vi "AnalysisDisplay_171213.vi"(0 "TraceLength":dbl, 1 "Segments":bool, 2 "FullTrack":bool, 3 "FulltrackonBackgroundSegments":picture, 4 "BackgroundSegments":picture, 5 "NormalMouseBackground":picture, 6 "X":i32, 7 "Y":i32, 8 "i":i32, 9 "X in":i32[](array[numeric]), 10 "Angle":dbl, 11 "Y in":i32[](array[numeric]), 14 "FulltrackonNormalMouseBackground":picture) -> (12 "X out":i32[](array[numeric]), 13 "Y out":i32[](array[numeric]), 19 "AnalysisDisplayOutput":picture)   [LabVIEW 2016]
uses:
  Globaltracker.vi
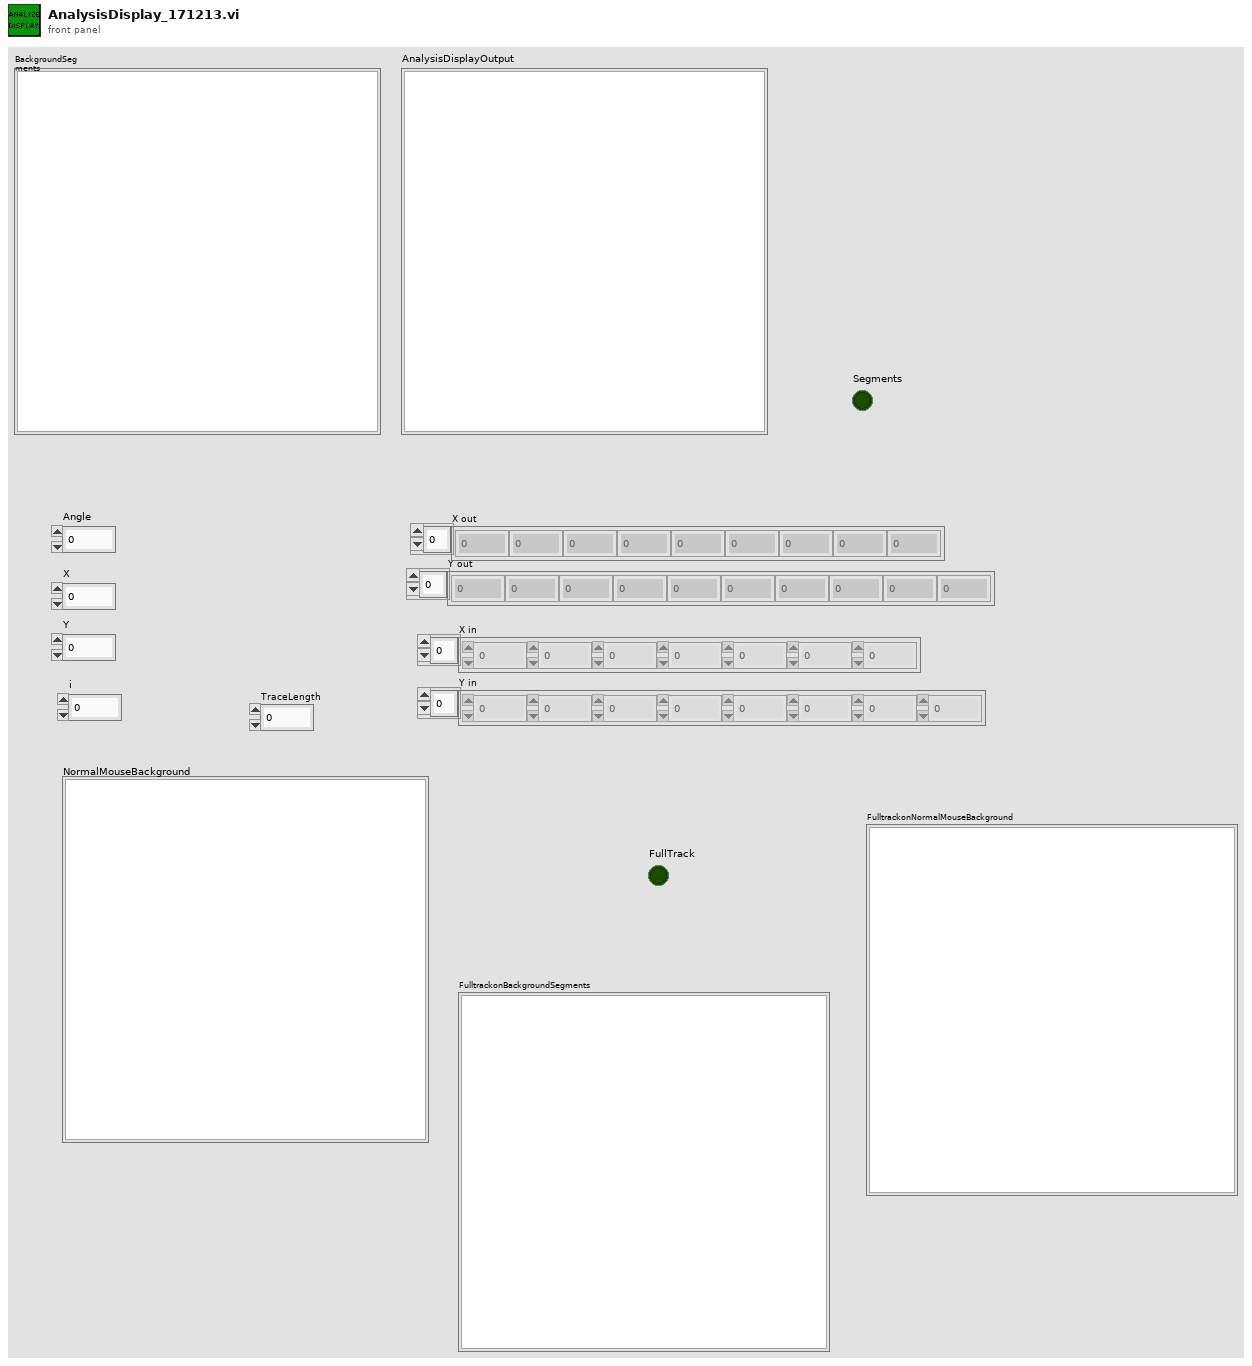
[diagram p1: front panel]
types:
  T1 = typedef "imagedata.ctl" = cluster{"image type":i32, "image depth":i32, "image":u8[], "mask":u8[], "colors":u32[], "Rectangle":cluster{"left":i16, "top":i16, "right":i16, "bottom":i16}}
  T2 = cluster{"left":i16, "top":i16, "right":i16, "bottom":i16}
  T3 = cluster{"image type":i32, "image depth":i32, "image":u8[], "mask":u8[], "colors":u32[], cluster{i32, i32, i32, i32}}
  T4 = cluster{"Width":u16, "Style":enum32{"Solid", "Dash", "Dot", "DashDot", "DashDotDot"}}
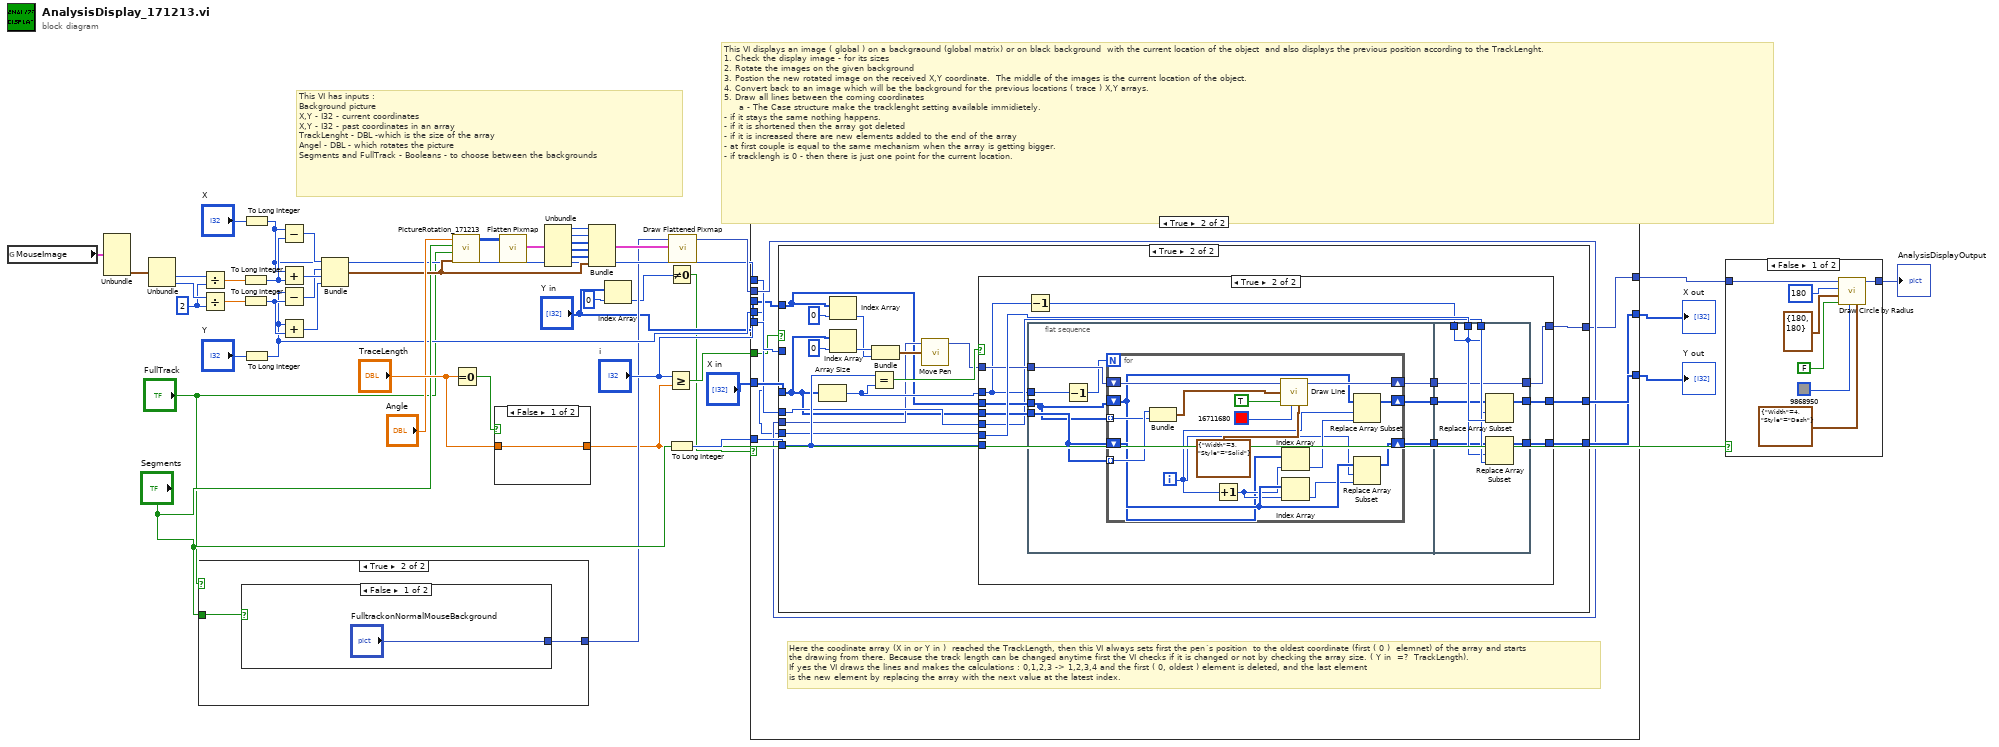
[diagram p0: block diagram]
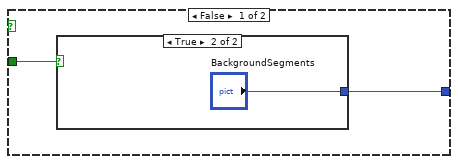
[diagram p2: hidden frame]
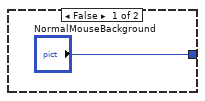
[diagram p3: hidden frame]
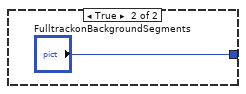
[diagram p4: hidden frame]
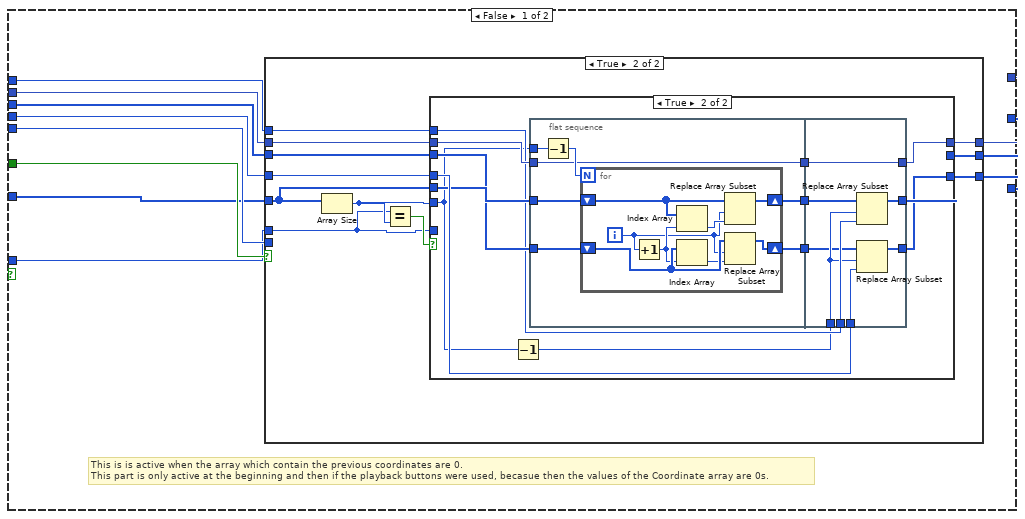
[diagram p5: hidden frame]
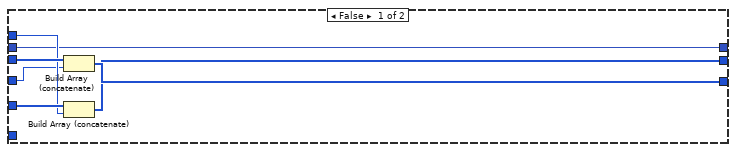
[diagram p6: hidden frame]
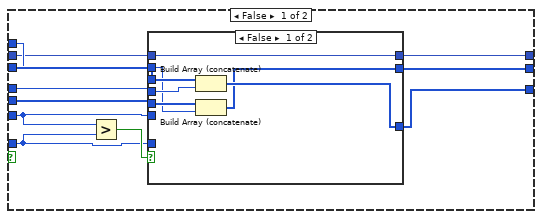
[diagram p7: hidden frame]
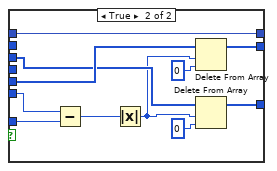
[diagram p8: hidden frame]
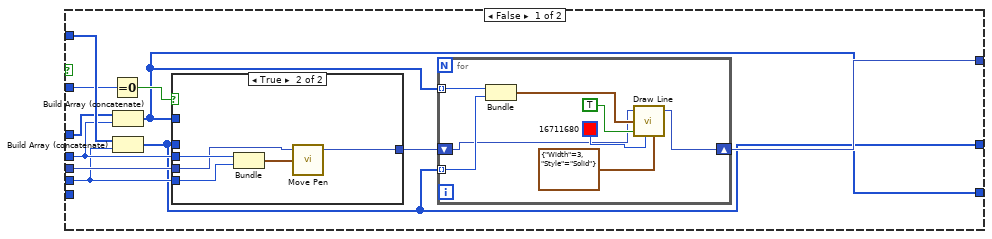
[diagram p9: hidden frame]
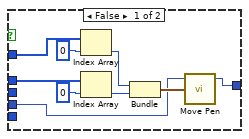
[diagram p10: hidden frame]
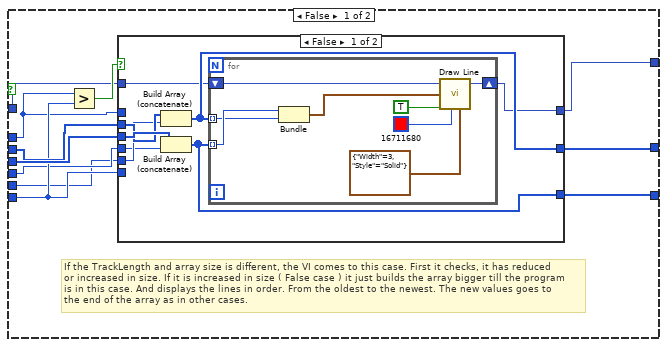
[diagram p11: hidden frame]
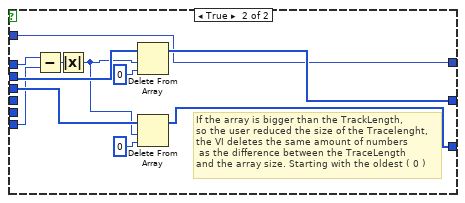
[diagram p12: hidden frame]
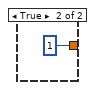
[diagram p13: hidden frame]
diagram:
  w19 = i16 2 ("y")
  # "This VI displays an image ( global ) on a backgraound (global matrix) or on black background  with the current location of the object  and also displays the previous position according to the TrackLenght.\n1. Check the display image - for its sizes\n2. Rotate the images on the given background\n3. Postion the new rotated image on the received X,Y coordinate.  The middle of the images is the current location of the object.\n4. Convert back to an image which will be the background for the previous locations ( trace ) X,Y arrays. \n5. Draw all lines between the coming coordinates \n     a - The Case structure make the tracklenght setting available immidietely. \n- if it stays the same nothing happens.\n- if it is shortened then the array got deleted\n- if it is increased there are new elements added to the end of the array\n- at first couple is equal to the same mechanism when the array is getting bigger.\n- if tracklengh is 0 - then there is just one point for the current location."
  # "This VI has inputs : \nBackground picture\nX,Y - I32 - current coordinates \nX,Y - I32 - past coordinates in an array \nTrackLenght - DBL -which is the size of the array\nAngel - DBL - which rotates the picture\nSegments and FullTrack - Booleans - to choose between the backgrounds"
  n1 = global read "Globaltracker.vi" "MouseImage"() -> (w23:T1)
  n2 = Unbundle(w23) -> ("Rectangle"=w22:T2)  [unwired: 5 out]
  n3 = Unbundle(w22) -> ("right"=w21:i16, "bottom"=w20:i16)  [unwired: 2 out]
  n4 = case shown="True" "FullTrack" {
    tunnel: "Segments" -> [w48 w52]
    tunnel: [w47 w51] -> w8
    frame False {
      n5 = case shown="True" w48 {
        tunnel: ["NormalMouseBackground" "BackgroundSegments"] -> w47
        frame False {
        }
        frame True {
        }
      }
    }
    frame True {
      n6 = case shown="False" w52 {
        tunnel: ["FulltrackonNormalMouseBackground" "FulltrackonBackgroundSegments"] -> w51
        frame False {
        }
        frame True {
        }
      }
    }
  }
  n7 = Divide(x=w21, y=w19) -> (x/y=w18:dbl)
  n8 = Divide(x=w20, y=w19) -> (x/y=w17:dbl)
  n9 = To Long Integer(number=w18) -> (32bit integer=w16:i32)
  n10 = To Long Integer(number=w17) -> (32bit integer=w15:i32)
  n11 = To Long Integer(number="X") -> (32bit integer=w10:i32)
  n12 = To Long Integer(number="Y") -> (32bit integer=w9:i32)
  n13 = Subtract(x=w10, y=w16) -> (x-y=w39:i32)
  n14 = Add(x=w10, y=w16) -> (x+y=w38:i32)
  n15 = Subtract(x=w9, y=w15) -> (x-y=w36:i32)
  n16 = Add(x=w9, y=w15) -> (x+y=w37:i32)
  n17 = Bundle(w39, w36, w38, w37) -> (w28:cluster{i32, i32, i32, i32})  [unwired: 1 in]
  n18 = call "PictureRotation_171213.vi"("Cluster"=w28, "FullTrack"="FullTrack", "Segments"="Segments", "Angle"="Angle") -> ("Array"=w14:u32[][])  [unwired: 7 in]
  n19 = Equal To 0?(x="TraceLength") -> (x = 0?=w45:bool)
  n20 = case shown="False" w45 {
    tunnel: "TraceLength" -> [w55 _]
    tunnel: [w55 1] -> w7
    frame False {
    }
    frame True {
    }
  }
  n21 = call <vilib>:"Flatten Pixmap.vi"("24-bit pixmap"=w14) -> ("image data"=w34:T1)  [unwired: 10 in]
  n22 = Unbundle(w34) -> ("image type"=w33:i32, "image depth"=w32:i32, "image"=w31:u8[], "mask"=w30:u8[], "colors"=w29:u32[])  [unwired: 1 out]
  n23 = Bundle("image type"=w33, "image depth"=w32, "image"=w31, "mask"=w30, "colors"=w29, w28) -> (w25:T3)  [unwired: 1 in]
  n24 = Index Array(array="Y in", index=0) -> (element=w4:i32)
  n25 = Greater Or Equal?(x="i", y=w7) -> (x >= y?=w6:bool)
  n26 = Not Equal To 0?(x=w4) -> (x != 0?=w3:bool)
  n27 = To Long Integer(number=w7) -> (32bit integer=w43:i32)
  n28 = call <vilib>:"Draw Flattened Pixmap.vi"("image data"=w25, "picture"=w8) -> ("new picture"=w24:picture)  [unwired: 7 in]
  n29 = case shown="True" w3 {
    tunnel: "i" -> [w66 w161]
    tunnel: w43 -> [w65 w160]
    tunnel: "X in" -> [w61 w159]
    tunnel: [w57 w158] -> w41
    tunnel: [w58 w157] -> w40
    tunnel: w24 -> [w60 w156]
    tunnel: [w59 w155] -> w13
    tunnel: w10 -> [w63 w154]
    tunnel: w9 -> [w64 w153]
    tunnel: "Y in" -> [w62 w152]
    tunnel: w6 -> [w67 w151]
    frame False {
      # "This is is active when the array which contain the previous coordinates are 0. \nThis part is only active at the beginning and then if the playback buttons were used, becasue then the values of the Coordinate array are 0s."
      n30 = case shown="True" w67 {
        tunnel: [w68 w84] -> w59
        tunnel: w66 -> [_ _]
        tunnel: w65 -> [_ w81]
        tunnel: w64 -> [w71 w80]
        tunnel: [w69 w78] -> w58
        tunnel: [w70 w85] -> w57
        tunnel: w62 -> [w74 w77]
        tunnel: w61 -> [w73 w76]
        tunnel: w63 -> [w72 w79]
        tunnel: w60 -> [w68 w75]
        frame False {
          n31 = Build Array (concatenate)(w74, w71) -> (w70:i32[])
          n32 = Build Array (concatenate)(w73, w72) -> (w69:i32[])
        }
        frame True {
          n33 = Array Size(array=w76) -> (size(s)=w82:i32)
          n34 = Equal?(x=w81, y=w82) -> (x = y?=w83:bool)
          n35 = case shown="True" w83 {
            tunnel: [w95 w127] -> w78
            tunnel: [w94 w126] -> w85
            tunnel: w80 -> [w86 w125]
            tunnel: w76 -> [w93 w124]
            tunnel: w77 -> [w92 w123]
            tunnel: w75 -> [w88 w122]
            tunnel: [w87 w118] -> w84
            tunnel: w82 -> [w90 w117]
            tunnel: w81 -> [w91 _]
            tunnel: w79 -> [w89 w121]
            frame False {
              n36 = Greater?(x=w90, y=w91) -> (0:w96:bool)
              n37 = case shown="False" w96 {
                tunnel: [w98 w114] -> w95
                tunnel: [w99 w113] -> w94
                tunnel: w93 -> [w103 w112]
                tunnel: w92 -> [w102 w111]
                tunnel: w90 -> [_ w110]
                tunnel: w91 -> [_ w106]
                tunnel: w86 -> [w101 _]
                tunnel: w89 -> [w100 _]
                tunnel: w88 -> [w97 w107]
                tunnel: [w97 w107] -> w87
                frame False {
                  n38 = Build Array (concatenate)(w102, w101) -> (w99:i32[])
                  n39 = Build Array (concatenate)(w103, w100) -> (w98:i32[])
                }
                frame True {
                  n40 = Subtract(x=w110, y=w106) -> (x-y=w109:i32)
                  n41 = Absolute Value(x=w109) -> (abs(x)=w108:i32)
                  n42 = Delete From Array(array=w112, length=w108, index=0) -> (array with subset deleted=w114:i32[])  [unwired: 1 out]
                  n43 = Delete From Array(array=w111, length=w108, index=0) -> (array with subset deleted=w113:i32[])  [unwired: 1 out]
                }
              }
            }
            frame True {
              n44 = Decrement(x=w117) -> (x-1=w120:i32)
              n45 = flat-sequence {
                tunnel: w124 -> [w134]
                tunnel: w123 -> [w133]
                tunnel: w122 -> [w128]
                tunnel: [w128] -> w119
                tunnel: w117 -> [w132]
                tunnel: [w130] -> w116
                tunnel: [w129] -> w115
                tunnel: [w150] -> w127
                tunnel: [w149] -> w126
                tunnel: w125 -> [w148]
                tunnel: w121 -> [w147]
                tunnel: w120 -> [w146]
                tunnel: w119 -> [w145]
                tunnel: [w145] -> w118
                tunnel: w116 -> [w144]
                tunnel: w115 -> [w143]
                frame #0 {
                  n46 = Decrement(x=w132) -> (x-1=w131:i32)
                  n47 = for {
                    N: w131 -> [_]
                    shift-right: [w136] -> w130
                    shift-left: w134 -> [w142]
                    shift-right: [w135] -> w129
                    shift-left: w133 -> [w141]
                    i -> [w137]
                    n48 = Increment(x=w137) -> (x+1=w140:i32)
                    n49 = Index Array(array=w142, index=w140) -> (element=w139:i32)
                    n50 = Index Array(array=w141, index=w140) -> (element=w138:i32)
                    n51 = Replace Array Subset(array=w142, new element=w139, index=w137) -> (w136:i32[])
                    n52 = Replace Array Subset(array=w141, new element=w138, index=w137) -> (w135:i32[])
                  }
                }
                frame #1 {
                  n53 = Replace Array Subset(array=w144, new element=w147, index=w146) -> (w150:i32[])
                  n54 = Replace Array Subset(array=w143, new element=w148, index=w146) -> (w149:i32[])
                }
              }
            }
          }
        }
      }
    }
    frame True {
      # "Here the coodinate array (X in or Y in )  reached the TrackLength, then this VI always sets first the pen´s position  to the oldest coordinate (first ( 0 )  elemnet) of the array and starts \nthe drawing from there. Because the track length can be changed anytime first the VI checks if it is changed or not by checking the array size. ( Y in  =?  TrackLength).\nIf yes the VI draws the lines and makes the calculations : 0,1,2,3 -> 1,2,3,4 and the first ( 0, oldest ) element is deleted, and the last element\nis the new element by replacing the array with the next value at the latest index."
      n55 = case shown="True" w151 {
        tunnel: [w170 w210] -> w155
        tunnel: w161 -> [w165 _]
        tunnel: w160 -> [_ w207]
        tunnel: w153 -> [w167 w206]
        tunnel: [w162 w204] -> w157
        tunnel: [w163 w211] -> w158
        tunnel: w152 -> [w172 w196]
        tunnel: w159 -> [w171 w195]
        tunnel: w154 -> [w169 w205]
        tunnel: w156 -> [w168 w198]
        frame False {
          n56 = Equal To 0?(x=w165) -> (x = 0?=w166:bool)
          n57 = Build Array (concatenate)(w171, w169) -> (w162:i32[])
          n58 = Build Array (concatenate)(w172, w167) -> (w163:i32[])
          n59 = case shown="True" w166 {
            tunnel: w169 -> [_ w186]
            tunnel: w168 -> [w179 w185]
            tunnel: w167 -> [_ w184]
            tunnel: [w180 w182] -> w164
            tunnel: w163 -> [w178 _]
            tunnel: w162 -> [w177 _]
            frame False {
              n60 = Index Array(array=w177, index=0) -> (element=w174:i32)
              n61 = Index Array(array=w178, index=0) -> (element=w173:i32)
              n62 = Bundle(w174, w173) -> (w181:cluster{i32, i32})  [unwired: 1 in]
              n63 = call <vilib>:"Move Pen.vi"("new position"=w181, "picture"=w179) -> ("new picture"=w180:picture)  [unwired: 3 in]
            }
            frame True {
              n64 = Bundle(w186, w184) -> (w183:cluster{i32, i32})  [unwired: 1 in]
              n65 = call <vilib>:"Move Pen.vi"("new position"=w183, "picture"=w185) -> ("new picture"=w182:picture)  [unwired: 3 in]
            }
          }
          n66 = for {
            tunnel: w162 -> [w194] mode=indexing
            tunnel: w163 -> [w193] mode=indexing
            shift-right: [w188] -> w170
            shift-left: w164 -> [w187]
            n67 = Bundle(w194, w193) -> (w189:cluster{i32, i32})  [unwired: 1 in]
            n68 = call <vilib>:"Draw Line.vi"("picture"=w187, "end point"=w189, "absolute coordinates?(T)"=TRUE, "color(black)"=u32 16711680, "pen"=T4 {"Width"=3, "Style"=enum."Solid"}) -> ("new picture"=w188:picture)  [unwired: 4 in]
          }
        }
        frame True {
          n69 = Array Size(array=w195) -> (size(s)=w208:i32)
          n70 = Index Array(array=w196, index=0) -> (element=w201:i32)
          n71 = Index Array(array=w195, index=0) -> (element=w202:i32)
          n72 = Equal?(x=w207, y=w208) -> (x = y?=w209:bool)
          n73 = Bundle(w202, w201) -> (w203:cluster{i32, i32})  [unwired: 1 in]
          n74 = call <vilib>:"Move Pen.vi"("new position"=w203, "picture"=w198) -> ("new picture"=w197:picture)  [unwired: 3 in]
          n75 = case shown="True" w209 {
            tunnel: [w221 w262] -> w204
            tunnel: [w220 w261] -> w211
            tunnel: w206 -> [w212 w260]
            tunnel: w195 -> [w219 w259]
            tunnel: w196 -> [w218 w258]
            tunnel: w197 -> [w214 w257]
            tunnel: [w213 w253] -> w210
            tunnel: w208 -> [w216 w252]
            tunnel: w207 -> [w217 _]
            tunnel: w205 -> [w215 w256]
            frame False {
              # "If the TrackLength and array size is different, the VI comes to this case. First it checks, it has reduced\nor increased in size. If it is increased in size ( False case ) it just builds the array bigger till the program\nis in this case. And displays the lines in order. From the oldest to the newest. The new values goes to\nthe end of the array as in other cases."
              n76 = Greater?(x=w216, y=w217) -> (0:w222:bool)
              n77 = case shown="False" w222 {
                tunnel: [w225 w249] -> w221
                tunnel: [w226 w248] -> w220
                tunnel: w219 -> [w230 w247]
                tunnel: w218 -> [w229 w246]
                tunnel: w216 -> [_ w245]
                tunnel: w217 -> [_ w241]
                tunnel: w212 -> [w228 _]
                tunnel: w215 -> [w227 _]
                tunnel: w214 -> [w224 w242]
                tunnel: [w223 w242] -> w213
                frame False {
                  n78 = Build Array (concatenate)(w229, w228) -> (w226:i32[])
                  n79 = Build Array (concatenate)(w230, w227) -> (w225:i32[])
                  n80 = for {
                    tunnel: w225 -> [w238] mode=indexing
                    tunnel: w226 -> [w237] mode=indexing
                    shift-right: [w231] -> w223
                    shift-left: w224 -> [w233]
                    n81 = Bundle(w238, w237) -> (w232:cluster{i32, i32})  [unwired: 1 in]
                    n82 = call <vilib>:"Draw Line.vi"("picture"=w233, "end point"=w232, "absolute coordinates?(T)"=TRUE, "color(black)"=u32 16711680, "pen"=T4 {"Width"=3, "Style"=enum."Solid"}) -> ("new picture"=w231:picture)  [unwired: 4 in]
                  }
                }
                frame True {
                  # "If the array is bigger than the TrackLength,\nso the user reduced the size of the Tracelenght,\nthe VI deletes the same amount of numbers\n as the difference between the TraceLength \nand the array size. Starting with the oldest ( 0 )"
                  n83 = Subtract(x=w245, y=w241) -> (x-y=w244:i32)
                  n84 = Absolute Value(x=w244) -> (abs(x)=w243:i32)
                  n85 = Delete From Array(array=w246, length=w243, index=0) -> (array with subset deleted=w248:i32[])  [unwired: 1 out]
                  n86 = Delete From Array(array=w247, length=w243, index=0) -> (array with subset deleted=w249:i32[])  [unwired: 1 out]
                }
              }
            }
            frame True {
              n87 = Decrement(x=w252) -> (x-1=w255:i32)
              n88 = flat-sequence {
                tunnel: w259 -> [w268]
                tunnel: w258 -> [w267]
                tunnel: w257 -> [w270]
                tunnel: [w269] -> w254
                tunnel: w252 -> [w266]
                tunnel: [w264] -> w251
                tunnel: [w263] -> w250
                tunnel: [w294] -> w262
                tunnel: [w293] -> w261
                tunnel: w260 -> [w292]
                tunnel: w256 -> [w291]
                tunnel: w255 -> [w290]
                tunnel: w254 -> [w289]
                tunnel: [w289] -> w253
                tunnel: w251 -> [w288]
                tunnel: w250 -> [w287]
                frame #0 {
                  n89 = Decrement(x=w266) -> (x-1=w265:i32)
                  n90 = for {
                    N: w265 -> [_]
                    tunnel: w268 -> [w286] mode=indexing
                    tunnel: w267 -> [w285] mode=indexing
                    shift-right: [w280] -> w269
                    shift-left: w270 -> [w282]
                    shift-right: [w275] -> w264
                    shift-left: w268 -> [w279]
                    shift-right: [w274] -> w263
                    shift-left: w267 -> [w273]
                    i -> [w272]
                    n91 = Bundle(w286, w285) -> (w281:cluster{i32, i32})  [unwired: 1 in]
                    n92 = Increment(x=w272) -> (x+1=w278:i32)
                    n93 = call <vilib>:"Draw Line.vi"("picture"=w282, "end point"=w281, "absolute coordinates?(T)"=TRUE, "color(black)"=u32 16711680, "pen"=T4 {"Width"=3, "Style"=enum."Solid"}) -> ("new picture"=w280:picture)  [unwired: 4 in]
                    n94 = Index Array(array=w273, index=w278) -> (element=w276:i32)
                    n95 = Index Array(array=w279, index=w278) -> (element=w277:i32)
                    n96 = Replace Array Subset(array=w273, new element=w276, index=w272) -> (w274:i32[])
                    n97 = Replace Array Subset(array=w279, new element=w277, index=w272) -> (w275:i32[])
                  }
                }
                frame #1 {
                  n98 = Replace Array Subset(array=w287, new element=w292, index=w290) -> (w293:i32[])
                  n99 = Replace Array Subset(array=w288, new element=w291, index=w290) -> (w294:i32[])
                }
              }
            }
          }
        }
      }
    }
  }
  "Y out" <- w41
  "X out" <- w40
  n100 = case shown="False" "Segments" {
    tunnel: w13 -> [w299 w302]
    tunnel: [w298 w302] -> w12
    frame False {
      n101 = call <vilib>:"Draw Circle by Radius.vi"("pen"=T4 {"Width"=4, "Style"=enum."Dash"}, "color(black)"=u32 9868950, "fill?(F)"=FALSE, "pixel center"=cluster{"horizontal":i16, "vertical":i16} {"horizontal"=180, "vertical"=180}, "radius"=i16 180, "picture"=w299) -> ("new picture"=w298:picture)  [unwired: 5 in]
    }
    frame True {
    }
  }
  "AnalysisDisplayOutput" <- w12
